vi "Read movements.vi"(8 "error in (no error)":errorcluster, 10 "index":i32, 11 "MotorSim in":refnum<class "MotorSim.lvclass">) -> (0 "error out":errorcluster, 1 "period":u32, 2 "initial position (0)":i32, 3 "MotorSim out":refnum<class "MotorSim.lvclass">, 4 "translation (100)":i32, 5 "forward":bool)   [LabVIEW 2018, in "MotorSim.lvclass"]
uses:
  MotorSim.lvclass
  MotorSim.lvclass/MotorSim.ctl
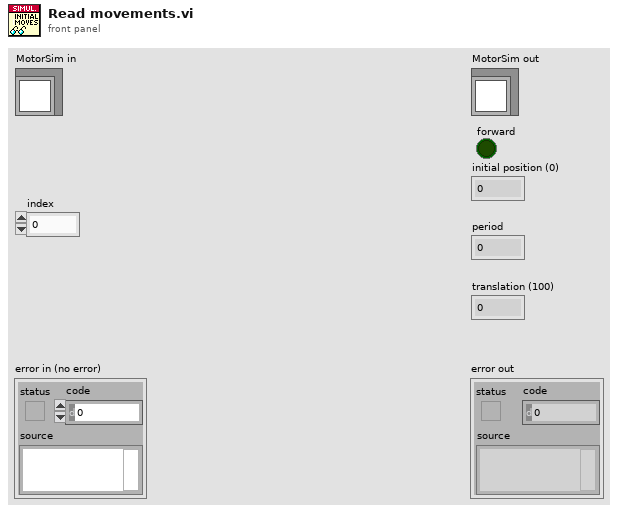
[diagram p1: front panel]
types:
  T1 = cluster{"period":u32, "initial position (0)":i32, "translation (100)":i32, "forward":bool}[]
  T2 = cluster{"period":u32, "initial position (0)":i32, "translation (100)":i32, "forward":bool}
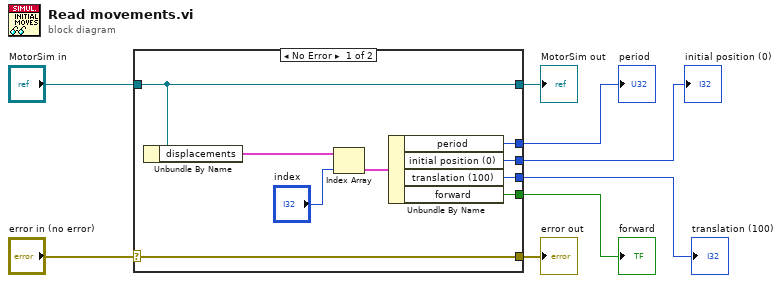
[diagram p0: block diagram]
diagram:
  n1 = case shown="No Error" "error in (no error)" {
    selector: "error in (no error)" -> [w17 w18]
    tunnel: [w17 w18] -> w7
    tunnel: [w16 w19] -> w5
    tunnel: "MotorSim in" -> [w16 w19]
    tunnel: [w12 _] -> w4
    tunnel: [w11 _] -> w3
    tunnel: [w10 _] -> w2
    tunnel: [w9 _] -> w1
    frame No Error {
      n2 = Unbundle By Name(w16) -> ("displacements"=w15:T1)
      n3 = Index Array(array=w15, index="index") -> (element=w13:T2)
      n4 = Unbundle By Name(w13) -> ("period"=w12:u32, "initial position (0)"=w11:i32, "translation (100)"=w10:i32, "forward"=w9:bool)
    }
    frame Error {
    }
  }
  "error out" <- w7
  "MotorSim out" <- w5
  "period" <- w4
  "initial position (0)" <- w3
  "translation (100)" <- w2
  "forward" <- w1
